vi "FlatToRichnixnet_grpc_DbRemoveAliasRequest.vi"(5 "OutputClusterType":T1, 11 "InputCluster":T2) -> (3 "OutputCluster":T1)   [LabVIEW 2025, in "xnet-grpc_client.lvlib"]
uses:
  nixnet_grpc_DbRemoveAliasRequest_Flat.ctl
  nixnet_grpc_DbRemoveAliasRequest.ctl
  xnet-grpc_client.lvlib
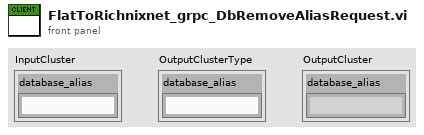
[diagram p1: front panel]
types:
  T1 = typedef "xnet-grpc_client.lvlib/nixnet_grpc_DbRemoveAliasRequest.ctl" = cluster{"database_alias":string}
  T2 = typedef "xnet-grpc_client.lvlib/nixnet_grpc_DbRemoveAliasRequest_Flat.ctl" = cluster{"database_alias":string}
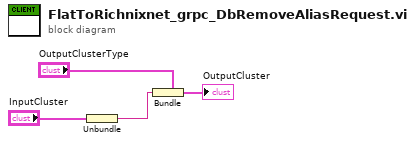
[diagram p0: block diagram]
diagram:
  n1 = Unbundle "Unbundle"("InputCluster") -> ("database_alias"=w1:string)
  n2 = Bundle "Bundle"(cluster="OutputClusterType", "database_alias"=w1) -> (→"OutputCluster":T1)
